vi "GlobalVariables.vi"() -> ()   [LabVIEW 2024]
panel:
  in  "nMotors 3":i32
  in  "whichMotors 3":i32[](array[numeric])
  in  "whichMotors 2":i32[](array[numeric])
  in  "whichMotors 1":i32[](array[numeric])
  in  "nMotors 1":i32
  in  "nMotors 2":i32
  in  "Period_LL":dbl
  in  "whichMotors":i32[](array[numeric])
  in  "nMotors":i32
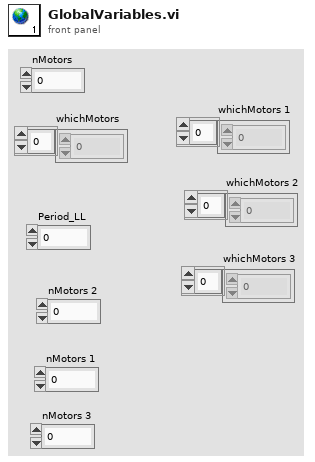
[diagram p1: front panel]
diagram:
